vi "test.vi"() -> ()   [LabVIEW 2020]
uses:
  <vilib>/Wiresmith Technology/G CLI/CLI Class/CLI.lvclass
panel:
  in  "VIs with # todo tasks":i32(listbox)
  in  "Fail on #todo items":bool
  out "num tests":i32
  in  "VIs Failed":i32(listbox)
  in  "VIs not loadable":i32(listbox)
  out "error type":enum16{"fatal", "non-fatal", "warning"}(ring)
  in  "VIs without test coverage":i32(listbox)
  out "error out":errorcluster
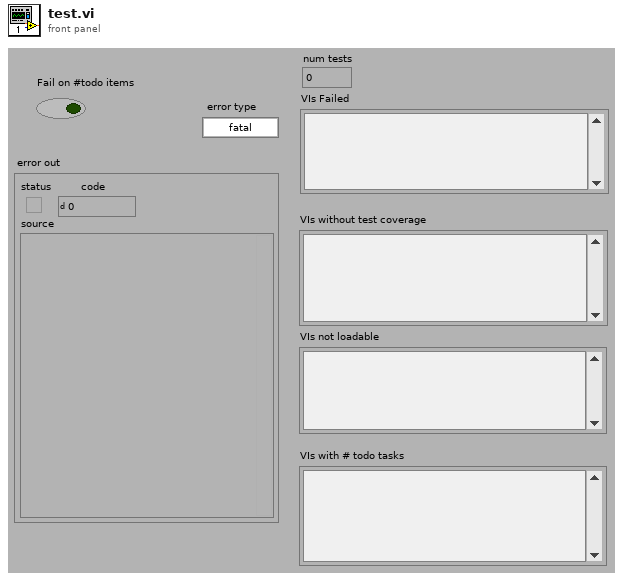
[diagram p1: front panel]
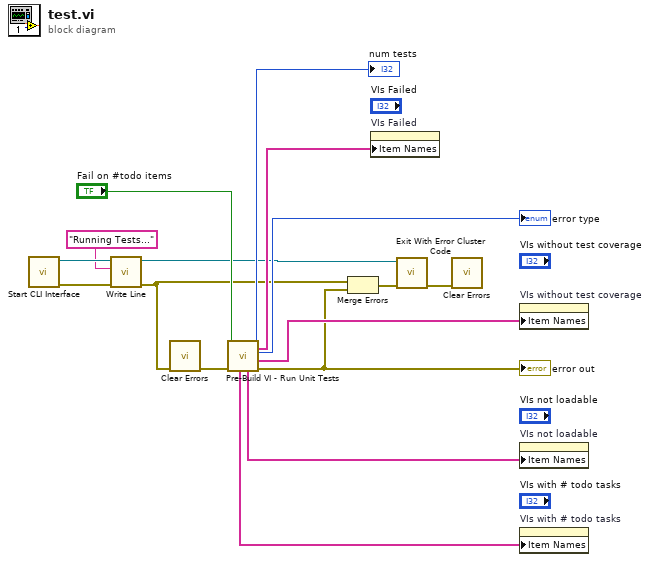
[diagram p0: block diagram]
diagram:
  n1 = call <vilib>:"Start CLI Interface.vi"() -> ("error out"=w9:errorcluster, "CLI out"=w8:refnum<class "CLI.lvclass">)  [unwired: 8 in, 2 out]
  n2 = call <vilib>:"Write Line.vi"("error in (no error)"=w9, "Text to Write"="Running Tests...", "CLI in"=w8) -> ("error out"=w2:errorcluster, "CLI out"=w5:refnum<class "CLI.lvclass">)  [unwired: 7 in]
  n3 = call <vilib>:"Clear Errors.vi"("error in (no error)"=w2) -> ("error out"=w4:errorcluster)  [unwired: 5 in, 1 out]
  n4 = call "Pre-Build VI - Run Unit Tests.vi"("error in (no error)"=w4, "Fail on #todo items"="Fail on #todo items") -> ("error out"=w6:errorcluster, "VIs without test coverage"=w16:string[], "error type"=→"error type":enum16{"fatal", "non-fatal", "warning"}, "num tests"=→"num tests":i32, "VIs not loadable"=w14:string[], "VIs Failed"=w13:string[], "VIs with #todo bookmarks"=w10:string[])  [unwired: 3 in]
  "error out" <- w6
  n5 = Merge Errors(w2, w6) -> (w3:errorcluster)
  n6 = property on="VIs Failed" class="LstBox (strict)"("Item Names"=w13) -> ()  [unwired: 2 in, 2 out]
  n7 = call <vilib>:"Exit With Error Cluster Code.vi"("error in (no error)"=w3, "CLI in"=w5) -> ("error out"=w1:errorcluster)  [unwired: 9 in]
  n8 = call <vilib>:"Clear Errors.vi"("error in (no error)"=w1) -> ()  [unwired: 5 in, 2 out]
  n9 = property on="VIs without test coverage" class="LstBox (strict)"("Item Names"=w16) -> ()  [unwired: 2 in, 2 out]
  n10 = property on="VIs not loadable" class="LstBox (strict)"("Item Names"=w14) -> ()  [unwired: 2 in, 2 out]
  n11 = property on="VIs with # todo tasks" class="LstBox (strict)"("Item Names"=w10) -> ()  [unwired: 2 in, 2 out]
